vi "DoughnutPlotExample1.vi"() -> ()   [LabVIEW 2019, in "HTMLPlot.lvclass"]
uses:
  HTMLPlot.lvclass
  Controls/LegendPosition.ctl
  Controls/PlotType.ctl
  Controls/GenericPlotOptions.ctl
  Controls/PiePlotOptions.ctl
  <vilib>/numeric/Random Number (Range) DBL.vi
  <vilib>/numeric/Random Number (Range) I64.vi
panel:
  in  "Graph 3":refnum<k7>(container)
  in  "Graph 2":refnum<k7>(container)
  out "error out":errorcluster
  in  "Graph":refnum<k7>(container)
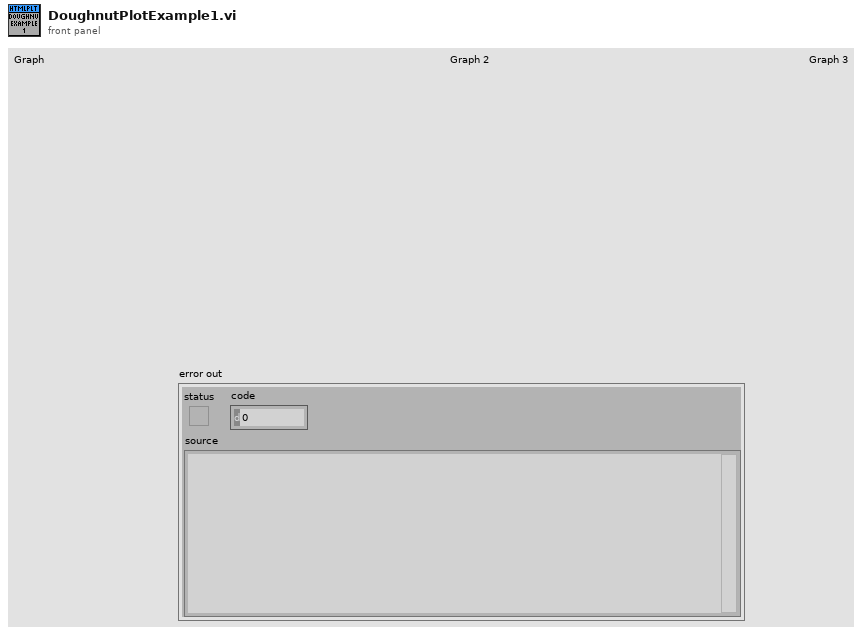
[diagram p1: front panel]
types:
  T1 = typedef "HTMLPlot.lvclass/PiePlotOptions.ctl" = cluster{"cutoutPercentage":i32}
  T2 = typedef "HTMLPlot.lvclass/GenericPlotOptions.ctl" = cluster{"GraphTitle":string, "LegendDisplay":bool, "LegendPosition":T3}
  T3 = typedef "HTMLPlot.lvclass/LegendPosition.ctl" = enum16{"top", "right", "left", "bottom"}
  T4 = typedef "HTMLPlot.lvclass/PlotType.ctl" = enum16{"bar", "line", "pie"}
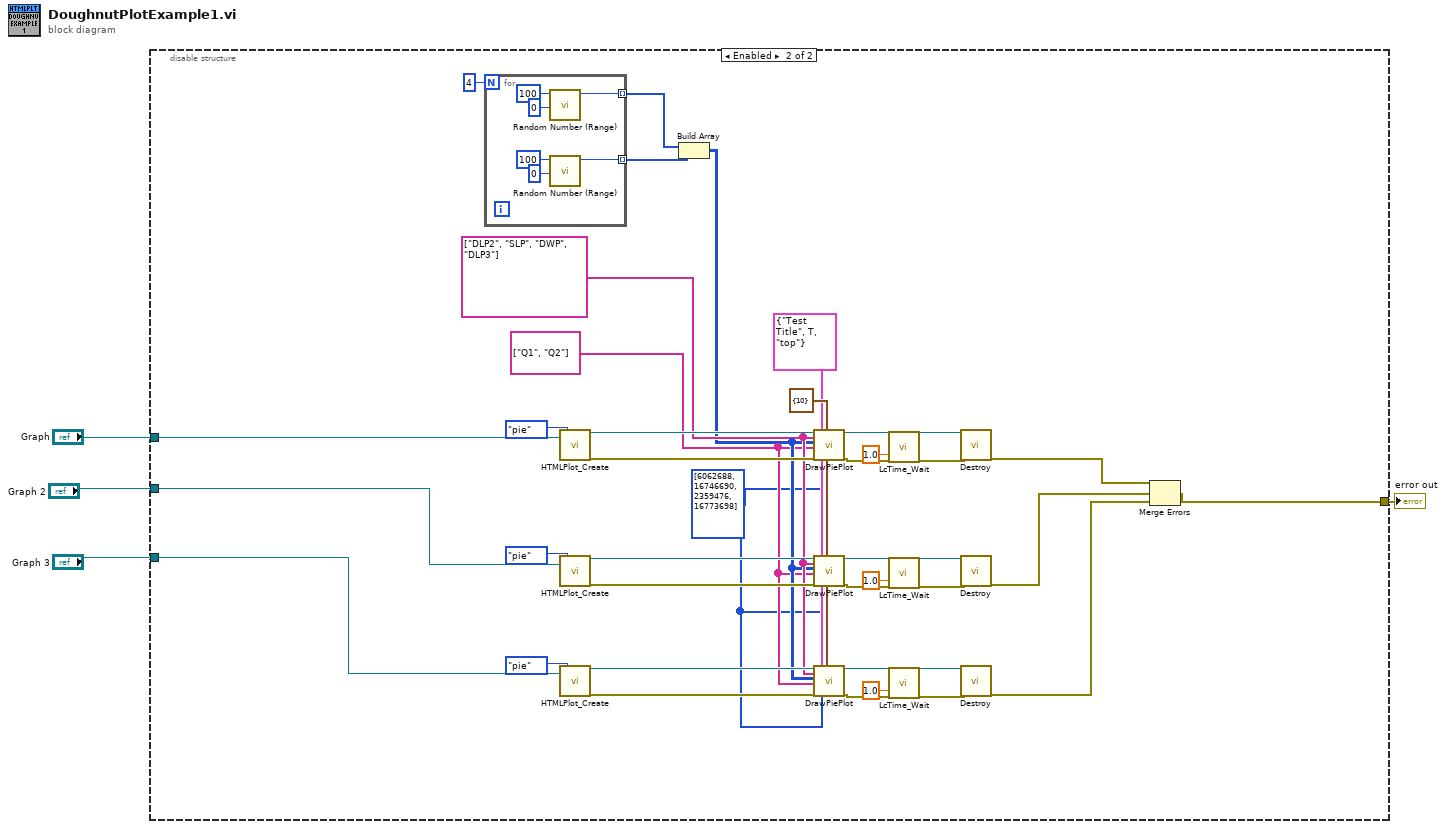
[diagram p0: block diagram]
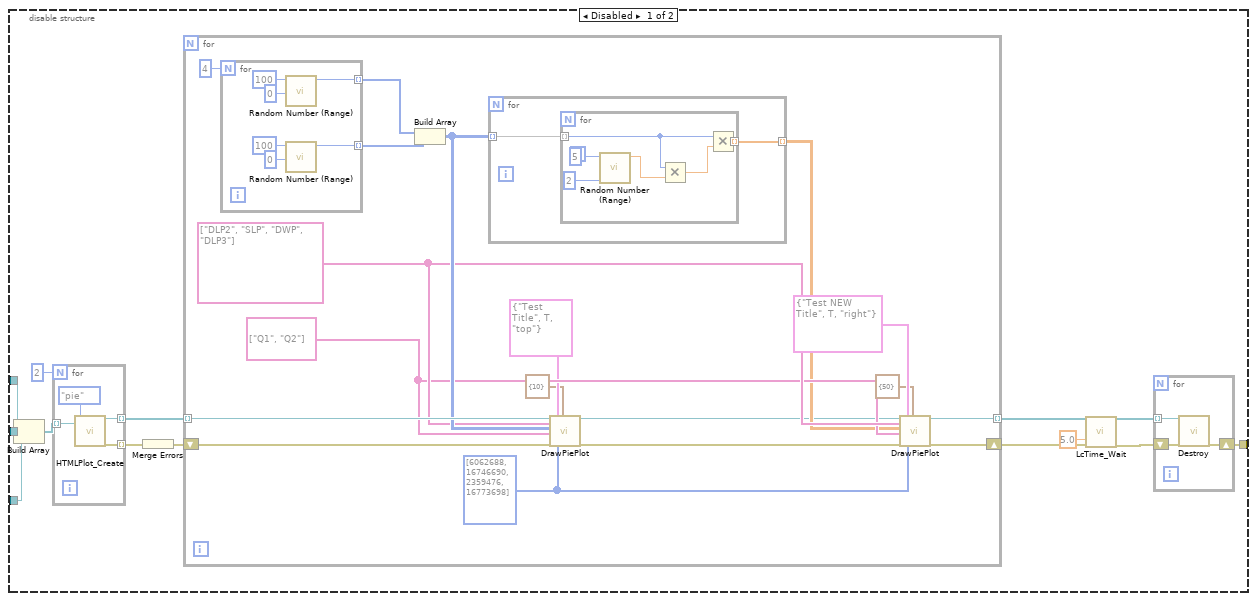
[diagram p2: hidden frame]
diagram:
  n1 = disable-structure shown="Enabled" {
    disable-tunnel: "Graph" -> [w15 w68]
    disable-tunnel: [w13 w60] -> w3
    disable-tunnel: "Graph 2" -> [w6 w67]
    disable-tunnel: "Graph 3" -> [w5 w66]
    frame Disabled {
      n2 = Build Array(w15, w6, w5) -> (w9:refnum<k7>[])
      n3 = for {
        N: 2 -> [_]
        tunnel: [w56] -> w17 mode=indexing
        tunnel: [w55] -> w16 mode=indexing
        tunnel: w9 -> [w53] mode=indexing
        n4 = call "HTMLPlot_Create.vi"("GraphContainer"=w53, "PlotType"=PlotType."pie" ("GenericProperties.PlotType")) -> ("reference out"=w56:refnum<class "HTMLPlot.lvclass">, "error out"=w55:errorcluster)  [unwired: 16 in]
      }
      n5 = Merge Errors(w16) -> (w8:errorcluster)
      n6 = for {
        tunnel: w17 -> [w38] mode=indexing
        tunnel: [w35] -> w14 mode=indexing
        shift-right: [w24] -> w12
        shift-left: w8 -> [w37]
        w32 = string[] ["Q1", "Q2"] ("PiePlot.PlotLabels")
        w36 = u32[] [6062688, 16746690, 2359476, 16773698] ("PlotColours")
        w33 = string[] ["DLP2", "SLP", "DWP", "DLP3"] ("DatasetLabels")
        n7 = for {
          N: 4 -> [_]
          tunnel: [w40] -> w22 mode=indexing
          tunnel: [w39] -> w21 mode=indexing
          n8 = call-poly <vilib>:"Random Number (Range).vi"("lower bound (-100)"=i64 0, "upper bound (100)"=i64 100) -> ("number"=w40:i64)  [unwired: 9 in]
          n9 = call-poly <vilib>:"Random Number (Range).vi"("lower bound (-100)"=i64 0, "upper bound (100)"=i64 100) -> ("number"=w39:i64)  [unwired: 9 in]
        }
        n10 = Build Array(w22, w21) -> (w34:i64[][])
        n11 = for {
          tunnel: w34 -> [w46] mode=indexing
          tunnel: [w45] -> w31 mode=indexing
          n12 = for {
            tunnel: w46 -> [w49] mode=indexing
            tunnel: [w52] -> w45 mode=indexing
            n13 = call-poly <vilib>:"Random Number (Range).vi"("lower bound (0)"=u64 2, "upper bound (100)"=u64 5) -> ("number"=w48:dbl)  [unwired: 9 in]
            n14 = Multiply(x=w49, y=w48) -> (x*y=w47:dbl)
            n15 = Multiply(x=w49, y=w47) -> (x*y=w52:dbl)
          }
        }
        n16 = call "DrawPiePlot.vi"("reference in"=w38, "PiePlot.PlotLabels"=w33, "PiePlot.Dataset"=w34, "PiePlot.DatasetLabels"=w32, "error in (no error)"=w37, "GenericPlotOptions"=T2 {"GraphTitle"="Test  Title", "LegendDisplay"=TRUE, "LegendPosition"=enum."top"}, "PiePlot.PlotColours"=w36, "PiePlotOptions"=T1 {"cutoutPercentage"=10}) -> ("reference out"=w30:refnum<class "HTMLPlot.lvclass">, "error out"=w29:errorcluster)  [unwired: 10 in]
        n17 = call "DrawPiePlot.vi"("reference in"=w30, "PiePlot.PlotLabels"=w33, "PiePlot.Dataset"=w31, "PiePlot.DatasetLabels"=w32, "error in (no error)"=w29, "GenericPlotOptions"=T2 {"GraphTitle"="Test NEW Title", "LegendDisplay"=TRUE, "LegendPosition"=enum."right"}, "PiePlot.PlotColours"=w36, "PiePlotOptions"=T1 {"cutoutPercentage"=50}) -> ("reference out"=w35:refnum<class "HTMLPlot.lvclass">, "error out"=w24:errorcluster)  [unwired: 10 in]
      }
      n18 = call "LcTime_Wait.vi"("secToWait"=5.0, "error in (no error)"=w12) -> ("error out"=w11:errorcluster)  [unwired: 15 in, 2 out]
      n19 = for {
        tunnel: w14 -> [w20] mode=indexing
        shift-right: [w19] -> w13
        shift-left: w11 -> [w18]
        n20 = call-dynamic "Destroy.vi"("reference in"=w20, "error in (no error)"=w18) -> ("error out"=w19:errorcluster)  [unwired: 16 in, 1 out]
      }
    }
    frame Enabled {
      w65 = T1 {"cutoutPercentage"=10} ("PiePlotOptions")
      w64 = T2 {"GraphTitle"="Test  Title", "LegendDisplay"=TRUE, "LegendPosition"=enum."top"} ("GenericPlotOptions")
      w61 = string[] ["Q1", "Q2"] ("PiePlot.PlotLabels")
      w57 = u32[] [6062688, 16746690, 2359476, 16773698] ("PlotColours")
      w63 = string[] ["DLP2", "SLP", "DWP", "DLP3"] ("DatasetLabels")
      n21 = for {
        N: 4 -> [_]
        tunnel: [w95] -> w92 mode=indexing
        tunnel: [w94] -> w91 mode=indexing
        n22 = call-poly <vilib>:"Random Number (Range).vi"("lower bound (-100)"=i64 0, "upper bound (100)"=i64 100) -> ("number"=w95:i64)  [unwired: 9 in]
        n23 = call-poly <vilib>:"Random Number (Range).vi"("lower bound (-100)"=i64 0, "upper bound (100)"=i64 100) -> ("number"=w94:i64)  [unwired: 9 in]
      }
      n24 = call "HTMLPlot_Create.vi"("GraphContainer"=w68, "PlotType"=PlotType."pie" ("GenericProperties.PlotType")) -> ("reference out"=w89:refnum<class "HTMLPlot.lvclass">, "error out"=w88:errorcluster)  [unwired: 16 in]
      n25 = call "HTMLPlot_Create.vi"("GraphContainer"=w67, "PlotType"=PlotType."pie" ("GenericProperties.PlotType")) -> ("reference out"=w77:refnum<class "HTMLPlot.lvclass">, "error out"=w78:errorcluster)  [unwired: 16 in]
      n26 = call "HTMLPlot_Create.vi"("GraphContainer"=w66, "PlotType"=PlotType."pie" ("GenericProperties.PlotType")) -> ("reference out"=w74:refnum<class "HTMLPlot.lvclass">, "error out"=w73:errorcluster)  [unwired: 16 in]
      n27 = Build Array(w92, w91) -> (w62:i64[][])
      n28 = call "DrawPiePlot.vi"("reference in"=w89, "PiePlot.PlotLabels"=w63, "PiePlot.Dataset"=w62, "PiePlot.DatasetLabels"=w61, "error in (no error)"=w88, "GenericPlotOptions"=w64, "PiePlot.PlotColours"=w57, "PiePlotOptions"=w65) -> ("reference out"=w84:refnum<class "HTMLPlot.lvclass">, "error out"=w87:errorcluster)  [unwired: 10 in]
      n29 = call "DrawPiePlot.vi"("reference in"=w77, "PiePlot.PlotLabels"=w63, "PiePlot.Dataset"=w62, "PiePlot.DatasetLabels"=w61, "error in (no error)"=w78, "GenericPlotOptions"=w64, "PiePlot.PlotColours"=w57, "PiePlotOptions"=w65) -> ("reference out"=w82:refnum<class "HTMLPlot.lvclass">, "error out"=w79:errorcluster)  [unwired: 10 in]
      n30 = call "DrawPiePlot.vi"("reference in"=w74, "PiePlot.PlotLabels"=w63, "PiePlot.Dataset"=w62, "PiePlot.DatasetLabels"=w61, "error in (no error)"=w73, "GenericPlotOptions"=w64, "PiePlot.PlotColours"=w57, "PiePlotOptions"=w65) -> ("reference out"=w69:refnum<class "HTMLPlot.lvclass">, "error out"=w72:errorcluster)  [unwired: 10 in]
      n31 = call "LcTime_Wait.vi"("secToWait"=1.0, "error in (no error)"=w87) -> ("error out"=w85:errorcluster)  [unwired: 15 in, 2 out]
      n32 = call "LcTime_Wait.vi"("secToWait"=1.0, "error in (no error)"=w79) -> ("error out"=w81:errorcluster)  [unwired: 15 in, 2 out]
      n33 = call "LcTime_Wait.vi"("secToWait"=1.0, "error in (no error)"=w72) -> ("error out"=w70:errorcluster)  [unwired: 15 in, 2 out]
      n34 = call-dynamic "Destroy.vi"("reference in"=w84, "error in (no error)"=w85) -> ("error out"=w83:errorcluster)  [unwired: 16 in, 1 out]
      n35 = call-dynamic "Destroy.vi"("reference in"=w82, "error in (no error)"=w81) -> ("error out"=w59:errorcluster)  [unwired: 16 in, 1 out]
      n36 = call-dynamic "Destroy.vi"("reference in"=w69, "error in (no error)"=w70) -> ("error out"=w58:errorcluster)  [unwired: 16 in, 1 out]
      n37 = Merge Errors(w83, w59, w58) -> (w60:errorcluster)
    }
  }
  "error out" <- w3
